vi "Janis_AC_4Channel_LKS331_6SRS830_SR5210_SR5110.vi"() -> ()   [LabVIEW 2014]
panel:
  out "PeakToPeak\nPiezoVoltage":dbl format="%#_13g"
  out "TimeStamp":dbl format="%#_13g"
  out "Y6":dbl
  out "X6":dbl
  out "Y5":dbl
  out "X5":dbl
  out "Y4":dbl
  out "X4":dbl
  out "Y3":dbl
  out "X3":dbl
  out "T2":dbl
  out "T1":dbl
  out "Y2":dbl
  out "Y1":dbl
  out "X2":dbl
  out "X1":dbl
  in  "Tab Control":T1(tab)
  in  "PiezoDrive":refnum<visa-resource-name>
  in  "PiezoGain":dbl
  in  "LKS Temp Controller":refnum<visa-resource-name>
  in  "Sample 2 V0":refnum<visa-resource-name>
  in  "Sample 1 V0":refnum<visa-resource-name>
  in  "SampleName":string
  in  "Sample \nThermometer":enum16{"T1", "T2"}(ring)
  in  "Sample 2 dV/dstrain":refnum<visa-resource-name>
  in  "Sample 1 dV/dstrain":refnum<visa-resource-name>
  in  "SG2 V0":refnum<visa-resource-name>
  in  "SG1 V0":refnum<visa-resource-name>
  out "TempAVsT":cluster{dbl, dbl}[](graph) caption="Temp Channel A"
  out "TempBvsT":cluster{dbl, dbl}[](graph) caption="Temp Channel B"
  in  "dV/dStrain:SG1 SR5110":string
  in  "dV/dStrain:SG2 SR5210":string
  out "X2":cluster{dbl, dbl}[](graph) caption="SRS1"
  out "X1":cluster{dbl, dbl}[](graph) caption="SRS1"
  out "Y1":cluster{dbl, dbl}[](graph) caption="SRS1"
  out "Y2":cluster{dbl, dbl}[](graph) caption="SRS1"
  out "X5":cluster{dbl, dbl}[](graph) caption="SRS1"
  out "Y5":cluster{dbl, dbl}[](graph) caption="SRS1"
  out "Y6":cluster{dbl, dbl}[](graph) caption="SRS1"
  out "X6":cluster{dbl, dbl}[](graph) caption="SRS1"
  out "X4":cluster{dbl, dbl}[](graph) caption="SRS1"
  out "Y4":cluster{dbl, dbl}[](graph) caption="SRS1"
  out "Y3":cluster{dbl, dbl}[](graph) caption="SRS1"
  out "X3 2":cluster{dbl, dbl}[](graph) caption="SRS1"
  out "X8":cluster{dbl, dbl}[](graph) caption="SRS1"
  out "Y8":cluster{dbl, dbl}[](graph) caption="SRS1"
  out "X7":cluster{dbl, dbl}[](graph) caption="SRS1"
  out "Y7":cluster{dbl, dbl}[](graph) caption="SRS1"
  out "Data is being stored here":string
  # "RealTime Data"
  # "INSTRUMENT ADDRESSES"
  # "Thermometry"
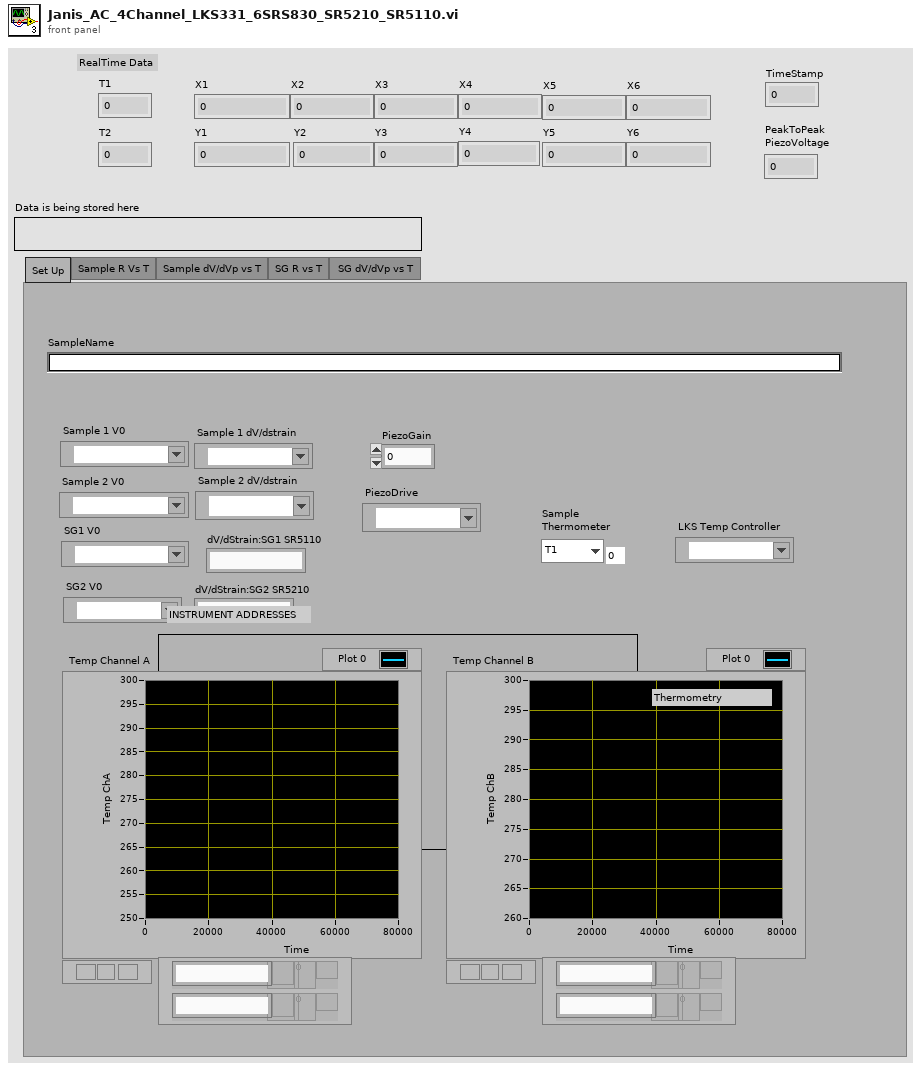
[diagram p1: front panel]
types:
  T1 = enum32{"Set Up", "Sample R Vs T", "Sample dV/dVp vs T", "SG R vs T", "SG dV/dVp vs T "}
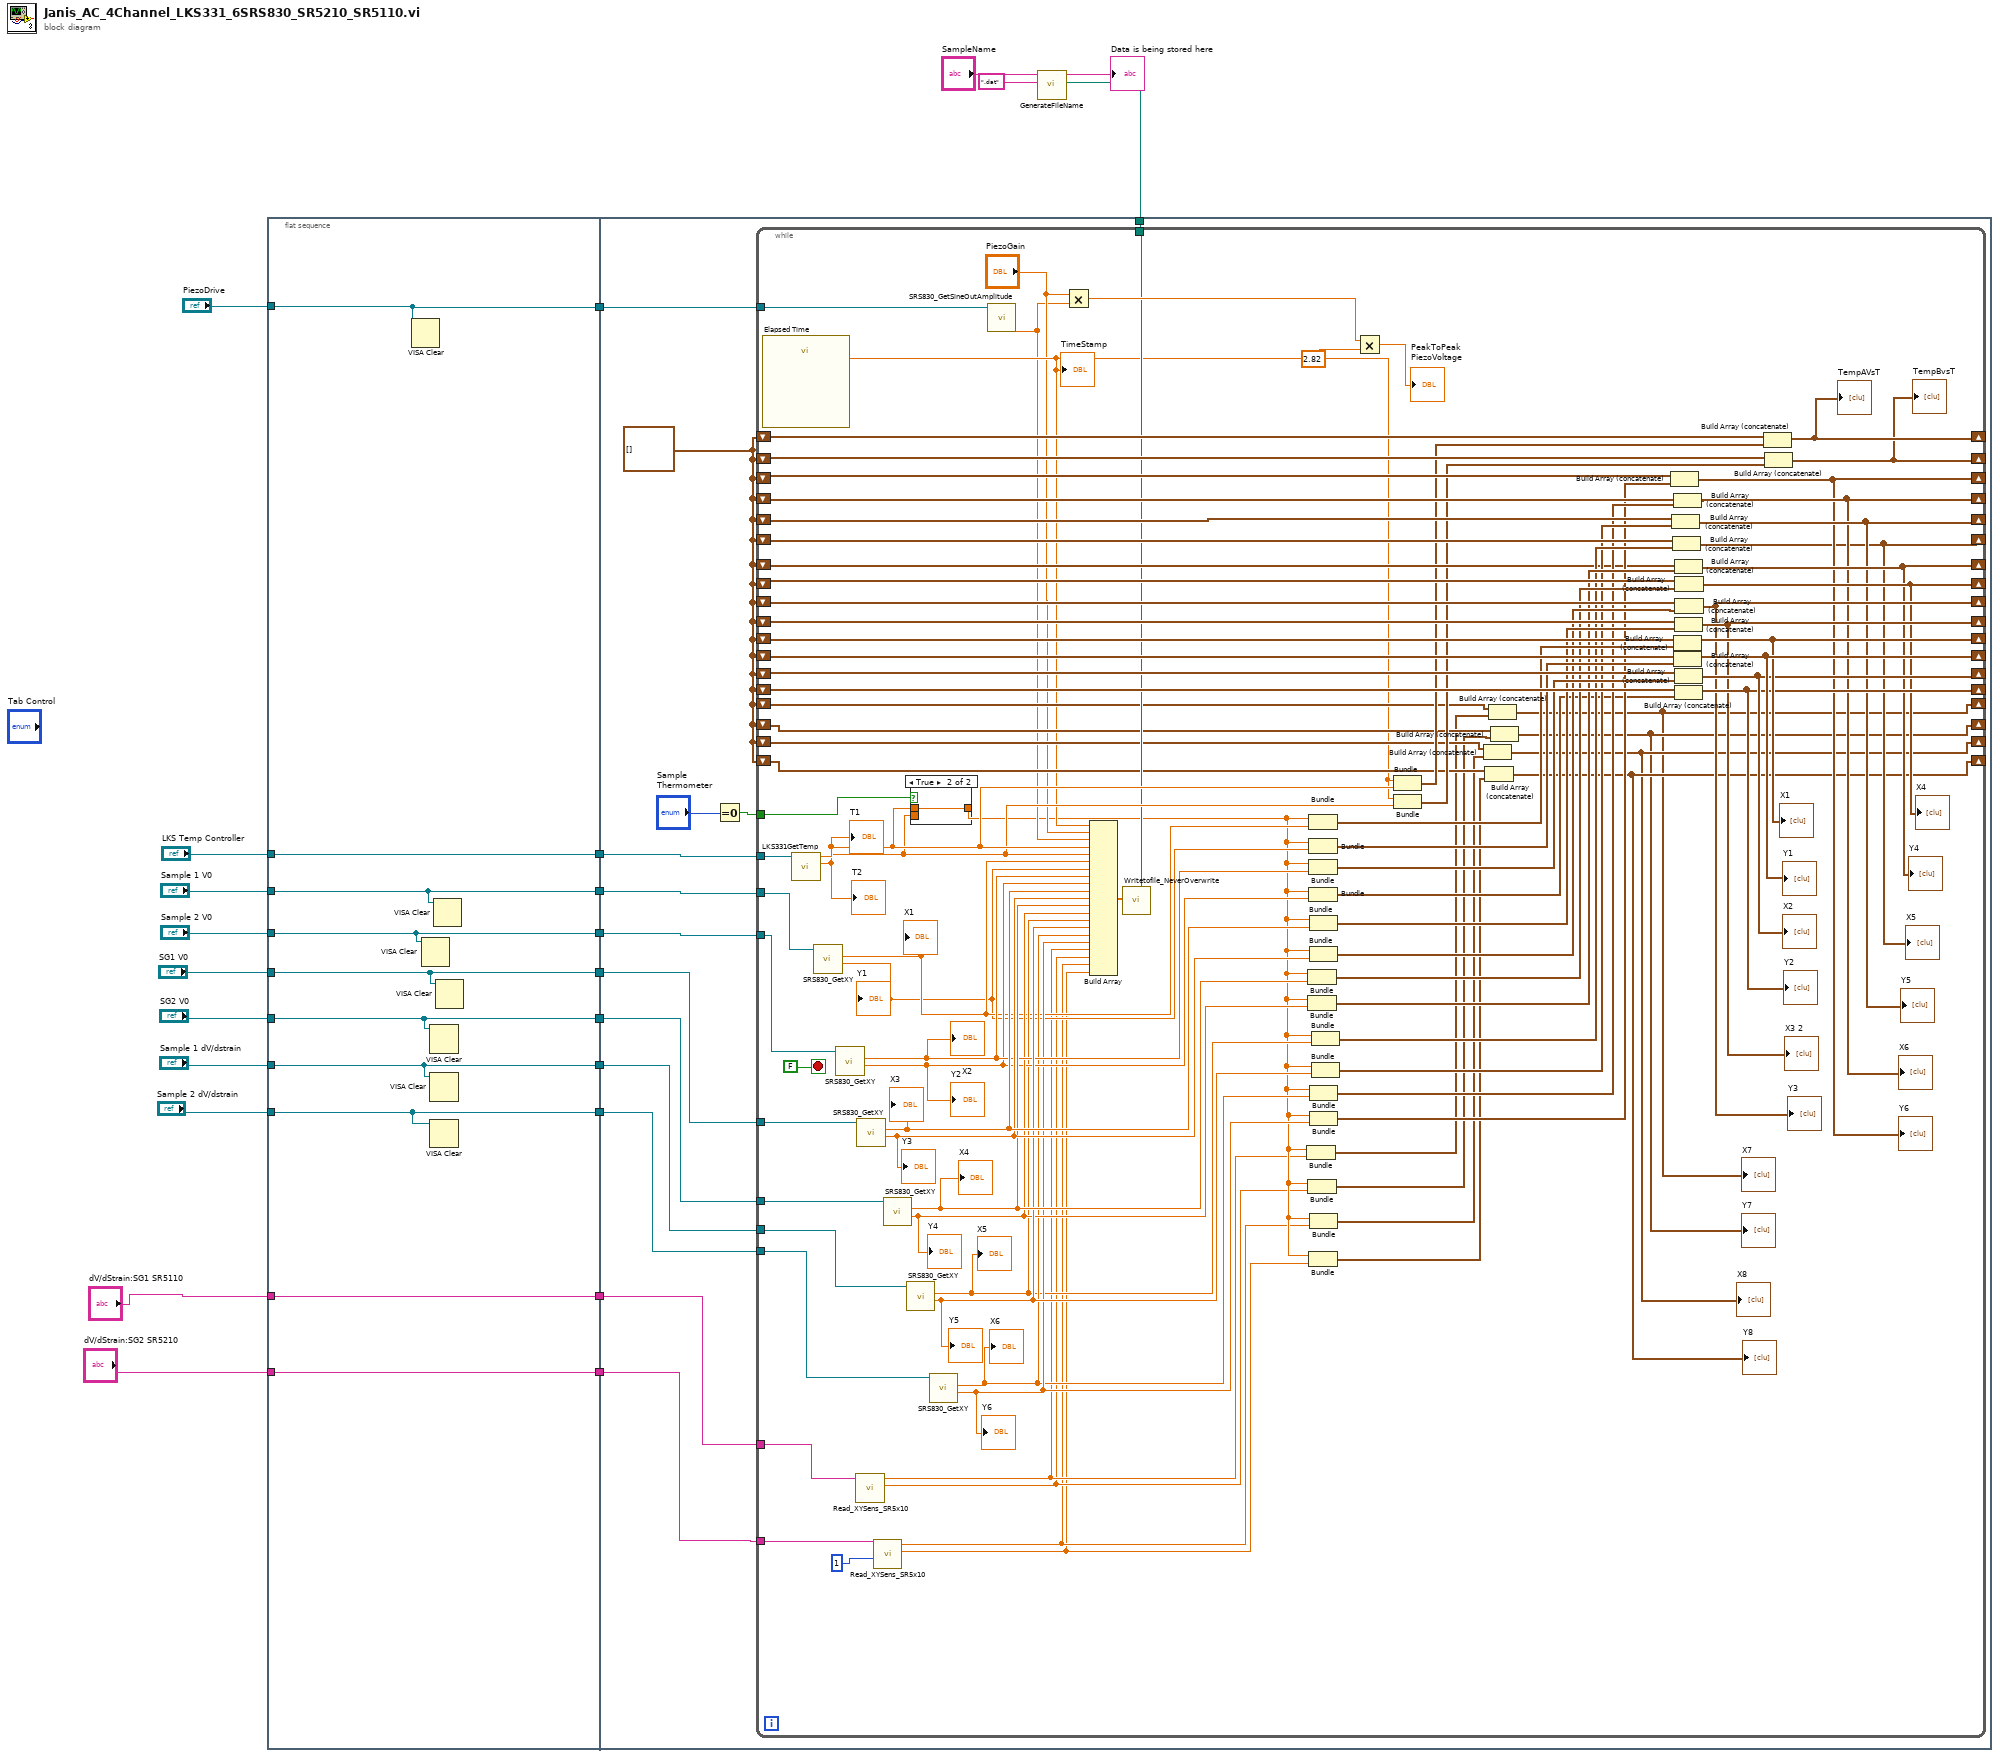
[diagram p0: block diagram]
diagram:
  n1 = flat-sequence {
    tunnel: "Sample 2 V0" -> [w31]
    tunnel: "Sample 1 V0" -> [w32]
    tunnel: "LKS Temp Controller" -> [w34]
    tunnel: [w34] -> w18
    tunnel: [w32] -> w17
    tunnel: [w31] -> w16
    tunnel: "SG1 V0" -> [w30]
    tunnel: [w30] -> w14
    tunnel: "SG2 V0" -> [w29]
    tunnel: [w29] -> w13
    tunnel: [w28] -> w12
    tunnel: "Sample 1 dV/dstrain" -> [w28]
    tunnel: [w33] -> w11
    tunnel: "Sample 2 dV/dstrain" -> [w33]
    tunnel: "PiezoDrive" -> [w27]
    tunnel: [w27] -> w6
    tunnel: [w25] -> w4
    tunnel: "dV/dStrain:SG2 SR5210" -> [w25]
    tunnel: [w26] -> w3
    tunnel: "dV/dStrain:SG1 SR5110" -> [w26]
    tunnel: w18 -> [w48]
    tunnel: w17 -> [w47]
    tunnel: w16 -> [w46]
    tunnel: w15 -> [w45]
    tunnel: w14 -> [w42]
    tunnel: w13 -> [w41]
    tunnel: w12 -> [w40]
    tunnel: w11 -> [w39]
    tunnel: w6 -> [w38]
    tunnel: w4 -> [w35]
    tunnel: w3 -> [w36]
    frame #0 {
      n2 = VISA Clear(VISA resource name=w27) -> ()  [unwired: 1 in, 2 out]
      n3 = VISA Clear(VISA resource name=w31) -> ()  [unwired: 1 in, 2 out]
      n4 = VISA Clear(VISA resource name=w29) -> ()  [unwired: 1 in, 2 out]
      n5 = VISA Clear(VISA resource name=w28) -> ()  [unwired: 1 in, 2 out]
      n6 = VISA Clear(VISA resource name=w33) -> ()  [unwired: 1 in, 2 out]
      n7 = VISA Clear(VISA resource name=w32) -> ()  [unwired: 1 in, 2 out]
      n8 = VISA Clear(VISA resource name=w30) -> ()  [unwired: 1 in, 2 out]
    }
    frame #1 {
      w37 = cluster{"T1":dbl, "Elapsed Time (s)":dbl}[] []
      n9 = Equal To 0?(x="Sample \nThermometer") -> (x = 0?=w44:bool)
      n10 = while {
        tunnel: w48 -> [w141]
        tunnel: w47 -> [w140]
        tunnel: w46 -> [w139]
        tunnel: w45 -> [w74]
        tunnel: w44 -> [w138]
        shift-right: [w125] -> _
        shift-left: w37 -> [w134]
        shift-right: [w124] -> _
        shift-left: w37 -> [w137]
        shift-right: [w127] -> _
        shift-left: w37 -> [w135]
        shift-right: [w126] -> _
        shift-left: w37 -> [w136]
        tunnel: w42 -> [w130]
        tunnel: w41 -> [w129]
        tunnel: w40 -> [w128]
        tunnel: w39 -> [w61]
        shift-right: [w105] -> _
        shift-left: w37 -> [w121]
        shift-right: [w103] -> _
        shift-left: w37 -> [w123]
        shift-right: [w102] -> _
        shift-left: w37 -> [w97]
        shift-right: [w104] -> _
        shift-left: w37 -> [w122]
        shift-right: [w99] -> _
        shift-left: w37 -> [w120]
        shift-right: [w100] -> _
        shift-left: w37 -> [w119]
        shift-right: [w101] -> _
        shift-left: w37 -> [w118]
        shift-right: [w96] -> _
        shift-left: w37 -> [w117]
        shift-right: [w80] -> _
        shift-left: w37 -> [w86]
        shift-right: [w79] -> _
        shift-left: w37 -> [w85]
        tunnel: w38 -> [w78]
        shift-right: [w49] -> _
        shift-left: w37 -> [w72]
        shift-right: [w50] -> _
        shift-left: w37 -> [w71]
        shift-right: [w51] -> _
        shift-left: w37 -> [w70]
        shift-right: [w52] -> _
        shift-left: w37 -> [w69]
        tunnel: w36 -> [w60]
        tunnel: w35 -> [w59]
        stop <- FALSE stop-if-true
        n11 = call "Elapsed Time"() -> ("Elapsed Time (s)"=w64:dbl)  [unwired: 12 in, 7 out]
        "TimeStamp" <- w64
        n12 = call "LKS331GetTemp.vi"("LKS Temp Controller"=w141) -> ("T2"=w83:dbl, "T1"=w84:dbl)  [unwired: 8 in, 1 out]
        "T1" <- w84
        "T2" <- w83
        n13 = call "SRS830_GetXY.vi"("SRS 830"=w140) -> ("Y"=w87:dbl, "X"=w88:dbl)  [unwired: 7 in, 2 out]
        "X1" <- w88
        "Y1" <- w87
        n14 = call "SRS830_GetXY.vi"("SRS 830"=w139) -> ("Y"=w92:dbl, "X"=w94:dbl)  [unwired: 7 in, 2 out]
        "X2" <- w94
        "Y2" <- w92
        n15 = call "Read_XYSens_SR5x10.vi"("7265 GPIB"=w60) -> ("Yout"=w55:dbl, "Xout"=w56:dbl)  [unwired: 8 in, 1 out]
        n16 = call "SRS830_GetXY.vi"("SRS 830"=w130) -> ("Y"=w115:dbl, "X"=w116:dbl)  [unwired: 7 in, 2 out]
        "X3" <- w116
        "Y3" <- w115
        n17 = call "Read_XYSens_SR5x10.vi"("Ring"=1, "7265 GPIB"=w59) -> ("Yout"=w53:dbl, "Xout"=w54:dbl)  [unwired: 7 in, 1 out]
        n18 = call "SRS830_GetXY.vi"("SRS 830"=w129) -> ("Y"=w93:dbl, "X"=w109:dbl)  [unwired: 7 in, 2 out]
        "X4" <- w109
        "Y4" <- w93
        n19 = call "SRS830_GetXY.vi"("SRS 830"=w128) -> ("Y"=w95:dbl, "X"=w89:dbl)  [unwired: 7 in, 2 out]
        "X5" <- w89
        "Y5" <- w95
        n20 = case shown="True" w138 {
          tunnel: w84 -> [_ w144]
          tunnel: w83 -> [w143 _]
          tunnel: [w143 w144] -> w57
          frame False {
          }
          frame True {
          }
        }
        n21 = call "SRS830_GetXY.vi"("SRS 830"=w61) -> ("Y"=w91:dbl, "X"=w90:dbl)  [unwired: 7 in, 2 out]
        "X6" <- w90
        "Y6" <- w91
        n22 = call "SRS830_GetSineOutAmplitude.vi"("VISA resource name"=w78) -> ("Measurement"=w62:dbl)  [unwired: 8 in, 2 out]
        n23 = Multiply(x="PiezoGain", y=w62) -> (x*y=w77:dbl)
        n24 = Build Array(w64, "PiezoGain", w62, w84, w83, w88, w87, w94, w92, w116, w115, w109, w93, w89, w95, w90, w91, w56, w55, w54, w53) -> (w73:dbl[])
        n25 = call "Writetofile_NeverOverwrite.vi"("appended array"=w73, "FilePathOut"=w74) -> ()  [unwired: 10 in]
        n26 = Bundle("T1"=w57, "Xout"=w56) -> (w65:cluster{"T1":dbl, "Xout":dbl})  [unwired: 1 in]
        n27 = Bundle("T1"=w57, "X"=w109) -> (w112:cluster{"T1":dbl, "X":dbl})  [unwired: 1 in]
        n28 = Bundle("T1"=w57, "Y"=w93) -> (w111:cluster{"T1":dbl, "Y":dbl})  [unwired: 1 in]
        n29 = Bundle("T1"=w57, "Yout"=w55) -> (w66:cluster{"T1":dbl, "Yout":dbl})  [unwired: 1 in]
        n30 = Bundle("T1"=w57, "X"=w88) -> (w133:cluster{"T1":dbl, "X":dbl})  [unwired: 1 in]
        n31 = Bundle("T1"=w57, "Y"=w87) -> (w132:cluster{"T1":dbl, "Y":dbl})  [unwired: 1 in]
        n32 = Bundle("T1"=w57, "X"=w94) -> (w131:cluster{"T1":dbl, "X":dbl})  [unwired: 1 in]
        n33 = Bundle("T1"=w57, "Y"=w92) -> (w98:cluster{"T1":dbl, "Y":dbl})  [unwired: 1 in]
        n34 = Bundle("T1"=w57, "Yout"=w53) -> (w68:cluster{"T1":dbl, "Yout":dbl})  [unwired: 1 in]
        n35 = Bundle("T1"=w57, "X"=w116) -> (w114:cluster{"T1":dbl, "X":dbl})  [unwired: 1 in]
        n36 = Bundle("T1"=w57, "Y"=w115) -> (w113:cluster{"T1":dbl, "Y":dbl})  [unwired: 1 in]
        n37 = Bundle("T1"=w57, "X"=w90) -> (w107:cluster{"T1":dbl, "X":dbl})  [unwired: 1 in]
        n38 = Bundle("T1"=w57, "Y"=w91) -> (w106:cluster{"T1":dbl, "Y":dbl})  [unwired: 1 in]
        n39 = Bundle("T1"=w57, "Xout"=w54) -> (w67:cluster{"T1":dbl, "Xout":dbl})  [unwired: 1 in]
        n40 = Bundle("T1"=w57, "X"=w89) -> (w110:cluster{"T1":dbl, "X":dbl})  [unwired: 1 in]
        n41 = Bundle("T1"=w57, "Y"=w95) -> (w108:cluster{"T1":dbl, "Y":dbl})  [unwired: 1 in]
        n42 = Multiply(x=w77, y=2.82) -> (x*y=→"PeakToPeak\nPiezoVoltage":dbl)
        n43 = Bundle("Elapsed Time (s)"=w64, "T1"=w84) -> (w81:cluster{"Elapsed Time (s)":dbl, "T1":dbl})  [unwired: 1 in]
        n44 = Bundle("Elapsed Time (s)"=w64, "T2"=w83) -> (w82:cluster{"Elapsed Time (s)":dbl, "T2":dbl})  [unwired: 1 in]
        n45 = Build Array (concatenate)(w70, w67) -> (w51:cluster{"T1":dbl, "Xout":dbl}[])
        "X8" <- w51
        n46 = Build Array (concatenate)(w69, w68) -> (w52:cluster{"T1":dbl, "Yout":dbl}[])
        "Y8" <- w52
        n47 = Build Array (concatenate)(w72, w65) -> (w49:cluster{"T1":dbl, "Xout":dbl}[])
        "X7" <- w49
        n48 = Build Array (concatenate)(w71, w66) -> (w50:cluster{"T1":dbl, "Yout":dbl}[])
        "Y7" <- w50
        n49 = Build Array (concatenate)(w120, w106) -> (w99:cluster{"T1":dbl, "Y":dbl}[])
        "Y6" <- w99
        n50 = Build Array (concatenate)(w118, w108) -> (w101:cluster{"T1":dbl, "Y":dbl}[])
        "Y5" <- w101
        n51 = Build Array (concatenate)(w117, w110) -> (w96:cluster{"T1":dbl, "X":dbl}[])
        "X5" <- w96
        n52 = Build Array (concatenate)(w119, w107) -> (w100:cluster{"T1":dbl, "X":dbl}[])
        "X6" <- w100
        n53 = Build Array (concatenate)(w136, w133) -> (w126:cluster{"T1":dbl, "X":dbl}[])
        "X1" <- w126
        n54 = Build Array (concatenate)(w135, w132) -> (w127:cluster{"T1":dbl, "Y":dbl}[])
        "Y1" <- w127
        n55 = Build Array (concatenate)(w97, w111) -> (w102:cluster{"T1":dbl, "Y":dbl}[])
        "Y4" <- w102
        n56 = Build Array (concatenate)(w121, w114) -> (w105:cluster{"T1":dbl, "X":dbl}[])
        "X3 2" <- w105
        n57 = Build Array (concatenate)(w134, w131) -> (w125:cluster{"T1":dbl, "X":dbl}[])
        "X2" <- w125
        n58 = Build Array (concatenate)(w137, w98) -> (w124:cluster{"T1":dbl, "Y":dbl}[])
        "Y2" <- w124
        n59 = Build Array (concatenate)(w123, w112) -> (w103:cluster{"T1":dbl, "X":dbl}[])
        "X4" <- w103
        n60 = Build Array (concatenate)(w122, w113) -> (w104:cluster{"T1":dbl, "Y":dbl}[])
        "Y3" <- w104
        n61 = Build Array (concatenate)(w86, w81) -> (w80:cluster{"Elapsed Time (s)":dbl, "T1":dbl}[])
        "TempAVsT" <- w80
        n62 = Build Array (concatenate)(w85, w82) -> (w79:cluster{"Elapsed Time (s)":dbl, "T2":dbl}[])
        "TempBvsT" <- w79
      }
    }
  }
  n63 = call "GenerateFileName.vi"("FileExtension"=".dat", "SampleName"="SampleName") -> ("FilePathOut"=w15:path, "FolderNameString"=→"Data is being stored here":string)  [unwired: 3 in, 1 out]
